vi "_ui.vi"() -> ()   [LabVIEW 2017, in "DebugConsole.lvlib"]
uses:
  DebugConsole.lvlib
panel:
  in  "Go":bool
  in  "Broadcast":string(combo)
  in  "1":string
  in  "SourceCSM":string(combo)
  in  "2":string
  in  "API":string(combo)
  in  "3":string
  in  "TargetCSM":string(combo)
  in  "Operation":T1(ring)
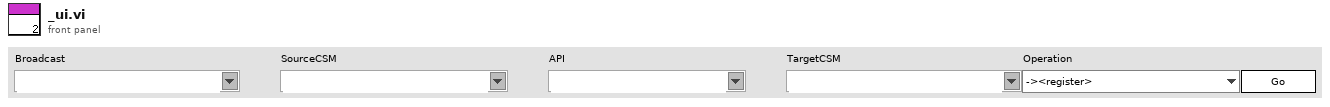
[diagram p1: front panel]
types:
  T1 = enum16{"-><register>", "-><register as status>", "-><register as interrupt>", "-><unregister>"}
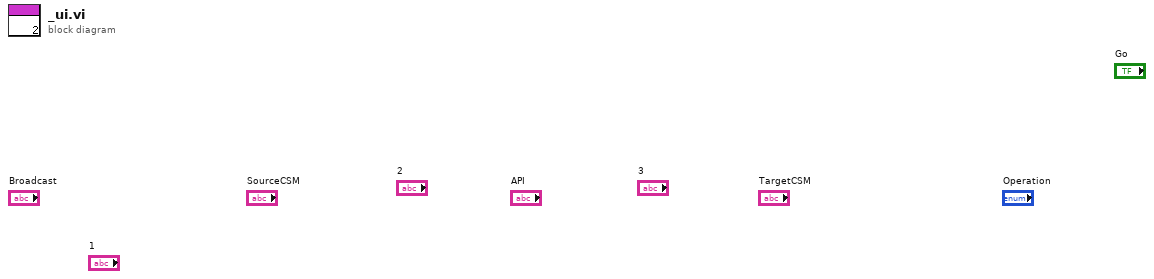
[diagram p0: block diagram]
diagram:
